vi "configure.vi"(8 "error in (no error)":errorcluster, 11 "CompactDAQ in":refnum<class "CompactDAQ.lvclass">) -> (0 "error out":errorcluster, 3 "CompactDAQ out":refnum<class "CompactDAQ.lvclass">)   [LabVIEW 2017, in "CompactDAQ.lvclass"]
uses:
  CompactDAQ.lvclass
  \\Mac\Home/Documents/MAL-Framework/user.lib/Common Components/Hardware/Hardware.lvclass
  <userlib>/Common Components/Hardware/Hardware.lvclass/Hardware.ctl
  <userlib>/Common Components/Hardware/DAQ/config/DAQ Configuration.lvclass
  <userlib>/Common Components/Hardware/DAQ/config/DAQ Configuration.lvclass/DAQ Configuration.ctl
  CompactDAQ.lvclass/CompactDAQ.ctl
  <vilib>/DAQmx/create/channels.llb/DAQmx Create Channel (AI-Voltage-Basic).vi
  <vilib>/DAQmx/configure/timing.llb/DAQmx Timing (Sample Clock).vi
  <userlib>/Common Components/Hardware/Hardware.lvclass
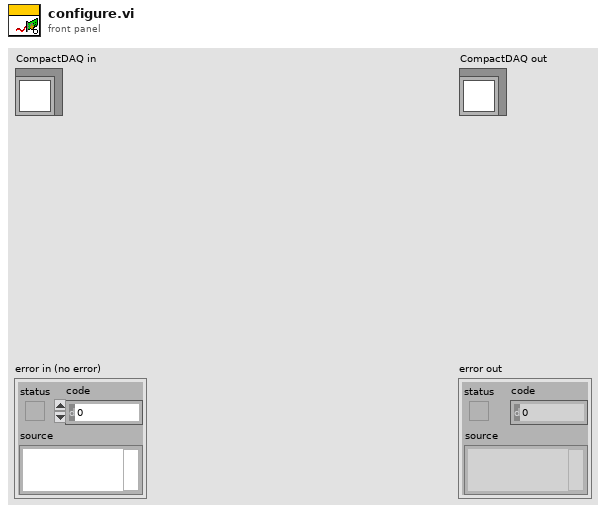
[diagram p1: front panel]
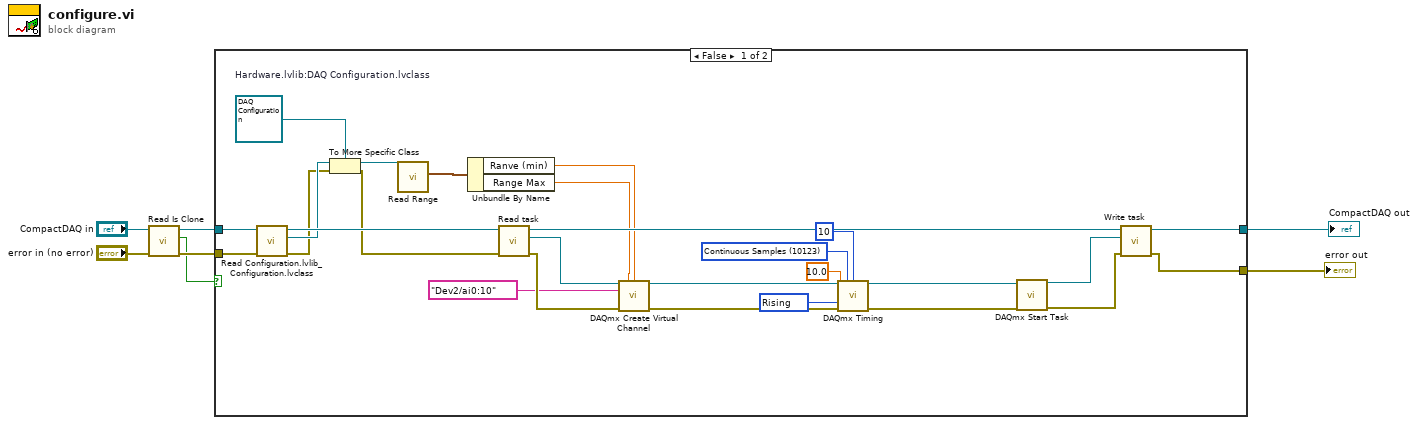
[diagram p0: block diagram]
diagram:
  n1 = call <userlib>:"Read Is Clone.vi"("error in (no error)"="error in (no error)", "Hardware in"="CompactDAQ in") -> ("error out"=w3:errorcluster, "Is Clone?"=w1:bool, "Hardware out"=w4:refnum<class "CompactDAQ.lvclass">)  [unwired: 7 in]
  n2 = case shown="False" w1 {
    tunnel: w4 -> [w18 w36]
    tunnel: w3 -> [w17 w35]
    tunnel: [w33 w36] -> w7
    tunnel: [w32 w35] -> w6
    frame False {
      w14 = refnum<class "DAQ Configuration.lvclass"> refnum  # Hardware.lvlib:DAQ Configuration.lvclass
      w21 = 10123 items=["Finite Samples"=10178, "Continuous Samples"=10123, "Hardware Timed Single Point"=12522] ("sample mode")
      w22 = 10280 items=["Rising"=10280, "Falling"=10171] ("active edge")
      n3 = call-dynamic "Read Configuration.lvlib_Configuration.lvclass.vi"("error in (no error)"=w17, "Hardware in"=w18) -> ("error out"=w13:errorcluster, "Hardware.lvlib:HW Configuration.lvclass"=w15:refnum<class "HW Configuration.lvclass">, "Hardware out"=w16:refnum<class "CompactDAQ.lvclass">)  [unwired: 7 in]
      n4 = To More Specific Class(target class=w14, reference=w15, error in=w13) -> (specific class reference=w11:refnum<class "DAQ Configuration.lvclass">, error out=w12:errorcluster)
      n5 = call <userlib>:"Read Range.vi"("DAQ Configuration in"=w11) -> ("Range"=w10:cluster{"Ranve (min)":dbl, "Range Max":dbl})  [unwired: 8 in, 2 out]
      n6 = Unbundle By Name(w10) -> ("Ranve (min)"=w8:dbl, "Range Max"=w9:dbl)
      n7 = call "Read task.vi"("error in (no error)"=w12, "CompactDAQ in"=w16) -> ("error out"=w28:errorcluster, "task"=w31:refnum<k21>, "CompactDAQ out"=w34:refnum<class "CompactDAQ.lvclass">)  [unwired: 7 in]
      n8 = call-poly <vilib>:"DAQmx Create Virtual Channel.vi"("task in"=w31, "maximum value"=w9, "minimum value"=w8, "physical channels"=tag "Dev2/ai0:10", "error in"=w28) -> ("task out"=w30:refnum<k21>, "error out"=w27:errorcluster)  [unwired: 9 in]
      n9 = call-poly <vilib>:"DAQmx Timing.vi"("task/channels in"=w30, "sample mode"=w21, "samples per channel"=10, "rate"=10.0, "active edge"=w22, "error in"=w27) -> ("task out"=w29:refnum<k21>, "error out"=w26:errorcluster)  [unwired: 8 in]
      n10 = call <vilib>:"DAQmx Start Task.vi"("task/channels in"=w29, "error in"=w26) -> ("task out"=w19:refnum<k21>, "error out"=w25:errorcluster)  [unwired: 12 in]
      n11 = call "Write task.vi"("error in (no error)"=w25, "task"=w19, "CompactDAQ in"=w34) -> ("error out"=w32:errorcluster, "CompactDAQ out"=w33:refnum<class "CompactDAQ.lvclass">)  [unwired: 7 in]
    }
    frame True {
    }
  }
  "error out" <- w6
  "CompactDAQ out" <- w7
